vi "HXG2_WriteTDMS.vi"(0 "Air-Liq Cluster":T3 {"Liq Cluster"."Liq TEMP %" min=0.0 max=100.0 step=1.0 format="%#.1f"; "Liq Cluster"."Liq FLOW %" min=0.0 max=100.0 step=1.0 format="%#.1f"; "Liq Cluster"."TLiq °F" min=40.0 max=180.0 step=1.0 format="%#.1f"; "Liq Cluster"."Mdot lbm/hr" min=0.0 max=1000.0 step=1.0 format="%#.1f"; "Air Cluster"."Air TEMP %" min=0.0 max=100.0 step=1.0 format="%#.1f"; "Air Cluster"."Air FLOW %" min=0.0 max=100.0 step=1.0 format="%#.1f"; "Air Cluster"."Tair  °F" min=-5.0 max=100.0 step=1.0 format="%#.1f"; "Air Cluster"."CFMs" min=0.0 max=200.0 step=1.0 format="%#.1f"}, 2 "Save?":bool, 5 "Calcs":T2, 7 "Excel/Elapsed t":dbl[](array[numeric]), 9 "DATA In":T1, 11 "error in":errorcluster, 12 "tdms file":refnum<k34>, 14 "Test Point":i32) -> (4 "tdms file out":refnum<k34>, 15 "error out":errorcluster)   [LabVIEW 2012]
uses:
  Controls/HXG2_AirGly-Cluster.ctl
  Controls/UI/HXG2_UI_ControlSetAir.ctl
  Controls/UI/HXG2_UI_ControlSetGly.ctl
  Controls/HXG2_Calculated.ctl
  Controls/HXG2_AnalogIn.ctl
  HXG2saveTimer.ctl
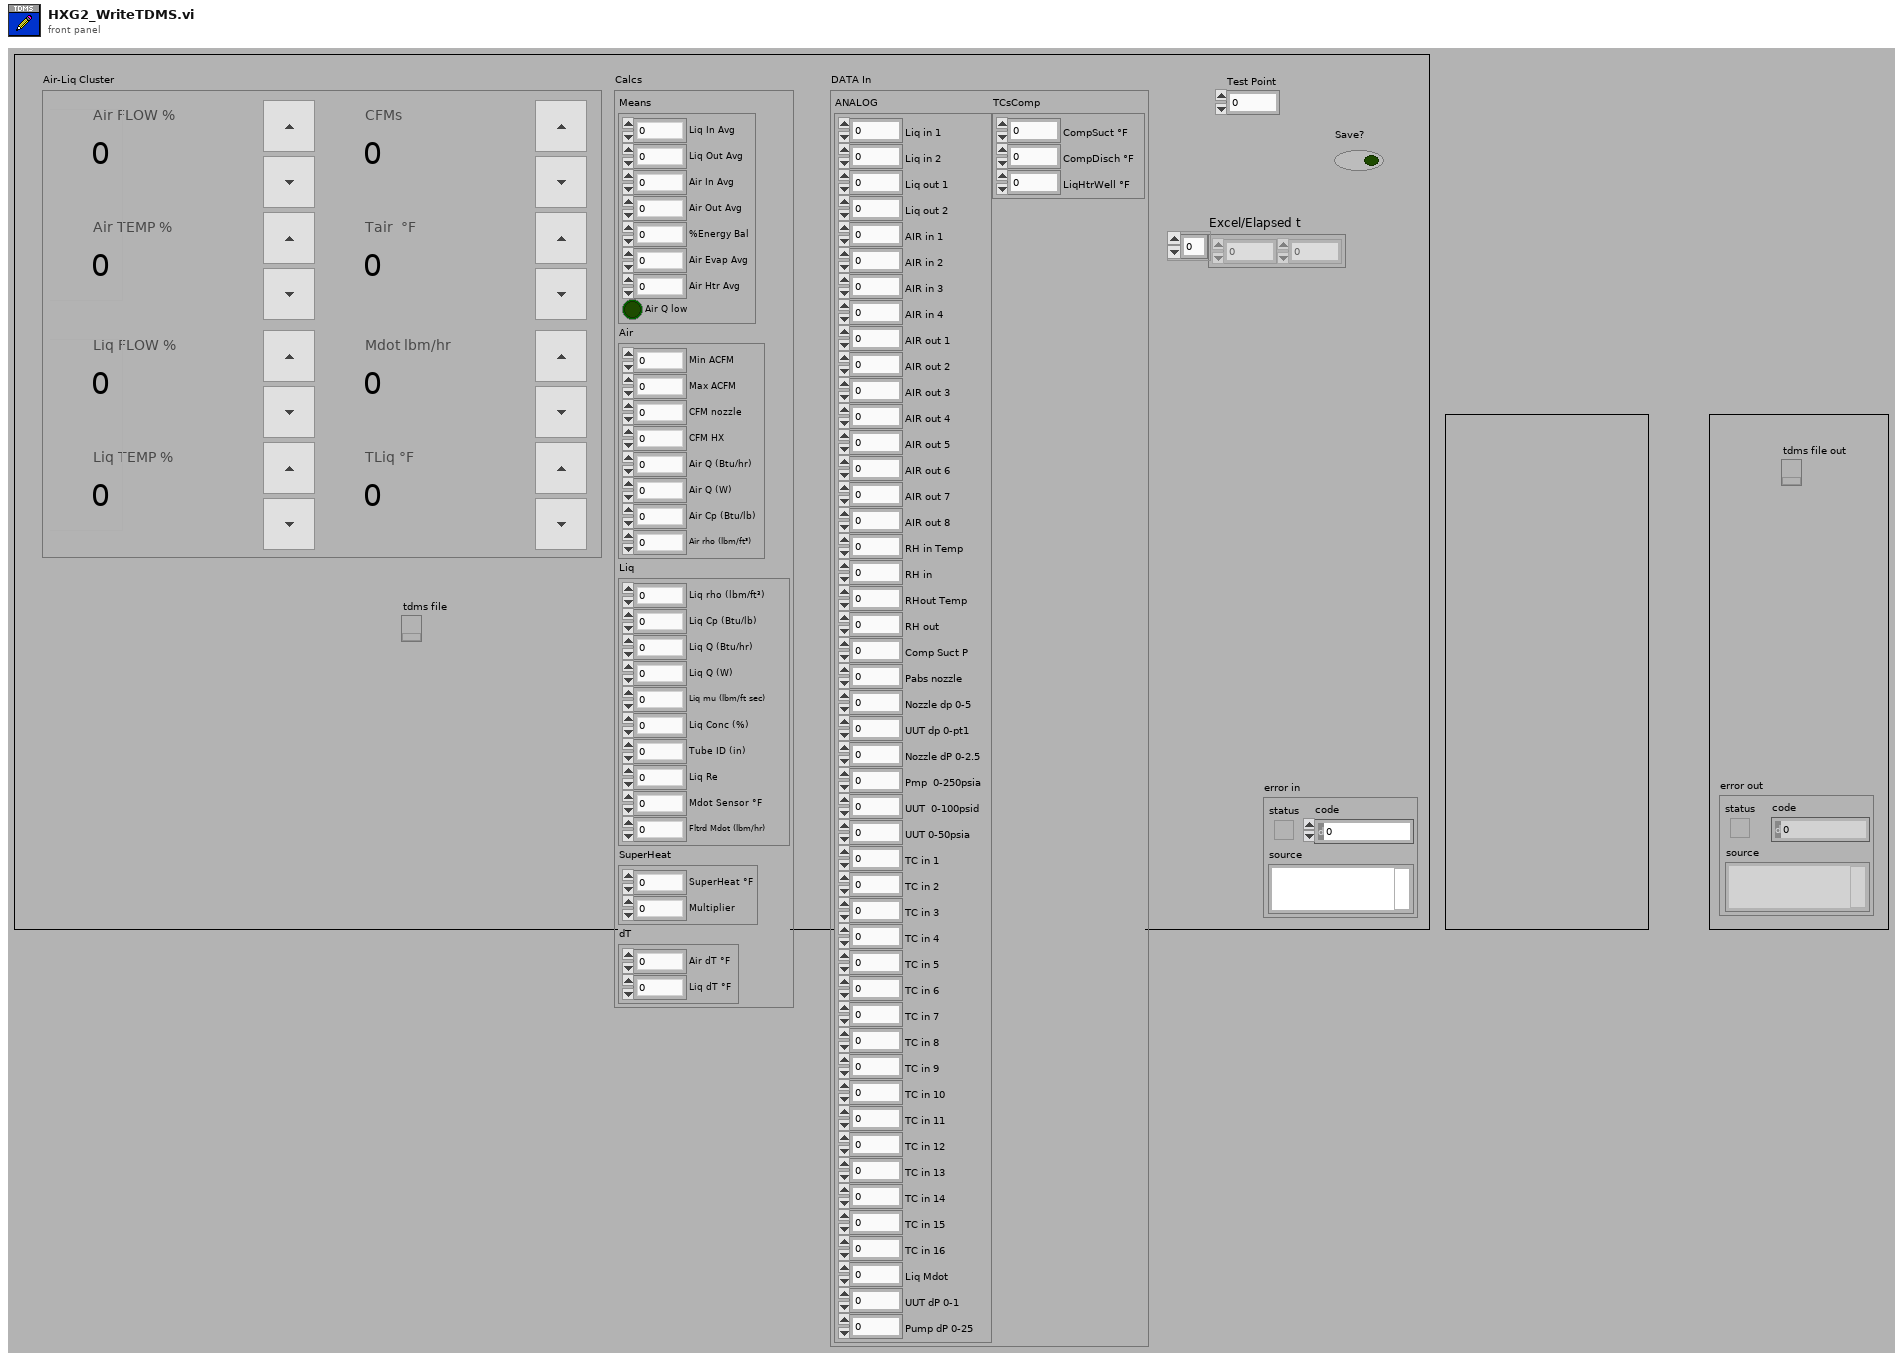
[diagram p1: front panel]
types:
  T1 = typedef "HXG2_AnalogIn.ctl" = cluster{"ANALOG":cluster{"Liq in 1":dbl, "Liq in 2":dbl, "Liq out 1":dbl, "Liq out 2":dbl, "AIR in 1":dbl, "AIR in 2":dbl, "AIR in 3":dbl, "AIR in 4":dbl, "AIR out 1":dbl, "AIR out 2":dbl, "AIR out 3":dbl, "AIR out 4":dbl, "AIR out 5":dbl, "AIR out 6":dbl, "AIR out 7":dbl, "AIR out 8":dbl, "RH in Temp":dbl, "RH in":dbl, "RHout Temp":dbl, "RH out":dbl, "Comp Suct P":dbl, "Pabs nozzle":dbl, "Nozzle dp 0-5":dbl, "UUT dp 0-pt1":dbl, "Nozzle dP 0-2.5":dbl, "Pmp  0-250psia":dbl, "UUT  0-100psid":dbl, "UUT 0-50psia":dbl, "TC in 1":dbl, "TC in 2":dbl, "TC in 3":dbl, "TC in 4":dbl, "TC in 5":dbl, "TC in 6":dbl, "TC in 7":dbl, "TC in 8":dbl, "TC in 9":dbl, "TC in 10":dbl, "TC in 11":dbl, "TC in 12":dbl, "TC in 13":dbl, "TC in 14":dbl, "TC in 15":dbl, "TC in 16":dbl, "Liq Mdot":dbl, "UUT dP 0-1":dbl, "Pump dP 0-25":dbl}, "TCsComp":cluster{"CompSuct °F  ":dbl, "CompDisch °F":dbl, "LiqHtrWell °F":dbl}}
  T2 = typedef "HXG2_Calculated.ctl" = cluster{"Means":cluster{"Liq In Avg":dbl, "Liq Out Avg":dbl, "Air In Avg":dbl, "Air Out Avg":dbl, "%Energy Bal":dbl, "Air Evap Avg":dbl, "Air Htr Avg":dbl, "Air Q low":bool}, "Air":cluster{"Min ACFM":dbl, "Max ACFM":dbl, "CFM nozzle":dbl, "CFM HX":dbl, "Air Q (Btu/hr)":dbl, "Air Q (W)":dbl, "Air Cp (Btu/lb)":dbl, "Air rho (lbm/ft³)":dbl}, "Liq":cluster{"Liq rho (lbm/ft³)":dbl, "Liq Cp (Btu/lb)":dbl, "Liq Q (Btu/hr)":dbl, "Liq Q (W)":dbl, "Liq mu (lbm/ft sec)":dbl, "Liq Conc (%)":dbl, "Tube ID (in)":dbl, "Liq Re":dbl, "Mdot Sensor °F":dbl, "Fltrd Mdot (lbm/hr)":dbl}, "SuperHeat":cluster{"SuperHeat °F":dbl, "Multiplier":dbl}, "dT":cluster{"Air dT °F":dbl, "Liq dT °F":dbl}}
  T3 = typedef "HXG2_AirGly-Cluster.ctl" = cluster{"Air Cluster":T4, "Liq Cluster":T5}
  T4 = typedef "HXG2_UI_ControlSetAir.ctl" = cluster{"Air FLOW %":dbl, "Air TEMP % ":dbl, "CFMs":dbl, "Tair  °F":dbl}
  T5 = typedef "HXG2_UI_ControlSetGly.ctl" = cluster{"Liq FLOW %":dbl, "Liq TEMP % ":dbl, "Mdot lbm/hr":dbl, "TLiq °F":dbl}
  T6 = typedef "HXG2saveTimer.ctl" = enum16{"EvntStrtDurtn", "EvntStrtInterv", "Stop", "Check", "RegStrtInterv", "Add10Durtn", "Take10Durtn"}
  T7 = cluster{"System Setpoints":string[], "Means":string[], "Air Props":string[], "Liq Props":string[], "System Data":string[], "All Temps":string[], "Other Data":string[], "CoilDesigner":string[]}
  T8 = typedef "HXG2_NumDisplayLarge.ctl" = dbl
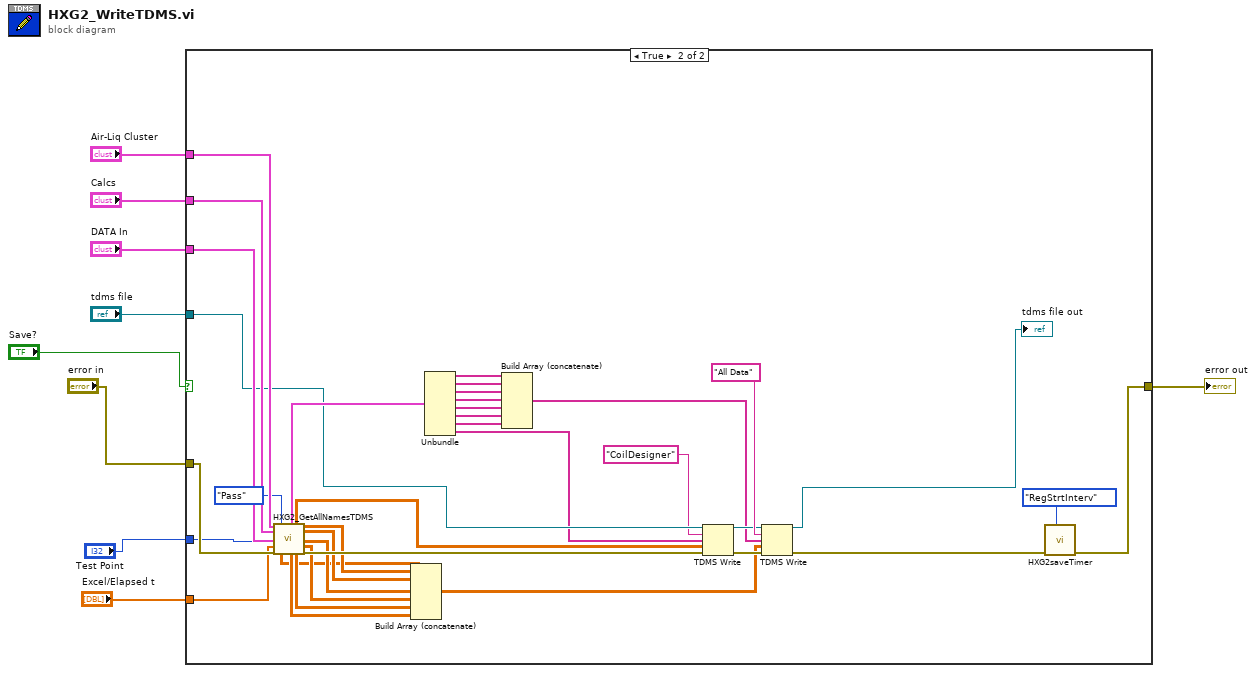
[diagram p0: block diagram]
diagram:
  n1 = case shown="True" "Save?" {
    tunnel: [w10 w32] -> w9
    tunnel: "Air-Liq Cluster" -> [_ w43]
    tunnel: "Calcs" -> [_ w42]
    tunnel: "DATA In" -> [_ w41]
    tunnel: "tdms file" -> [_ w36]
    tunnel: "error in" -> [w10 w35]
    tunnel: "Test Point" -> [_ w14]
    tunnel: "Excel/Elapsed t" -> [_ w13]
    frame False {
    }
    frame True {
      n2 = call "HXG2_GetAllNamesTDMS.vi"("Air-Liq Cluster"=w43, "Calcs"=w42, "DATA In"=w41, "Test Point"=w14, "Excel/Elapsed t"=w13, "error in (no error)"=w35, "Control"=enum16{"Initialize", "Pass"}."Pass") -> ("SetPoints"=w25:dbl[][], "Cluster"=w37:T7, "Other Data"=w26:dbl[][], "For CoilDesigner"=w38:T8[][], "All Temps"=w27:dbl[][], "Means"=w31:dbl[][], "Air Props"=w30:dbl[][], "Liq Props"=w29:dbl[][], "Syst Data"=w28:dbl[][], "error out"=w40:errorcluster)  [unwired: 3 in]
      n3 = Build Array (concatenate)(w25, w31, w30, w29, w28, w27, w26) -> (w24:dbl[][])
      n4 = Unbundle(w37) -> ("System Setpoints"=w22:string[], "Means"=w21:string[], "Air Props"=w20:string[], "Liq Props"=w19:string[], "System Data"=w18:string[], "All Temps"=w17:string[], "Other Data"=w16:string[], "CoilDesigner"=w23:string[])
      n5 = Build Array (concatenate)(w22, w21, w20, w19, w18, w17, w16) -> (w15:string[])
      n6 = TDMS Write(0:w36, 5:"CoilDesigner", 7:w23, 9:w38, 11:w40) -> (4:w44:refnum<k34>, 15:w45:errorcluster)  [unwired: 1 in, 2 out]
      n7 = TDMS Write(0:w44, 5:"All Data", 7:w15, 9:w24, 11:w45) -> (4:→"tdms file out":refnum<k34>, 15:w12:errorcluster)  [unwired: 1 in, 2 out]
      n8 = call "HXG2saveTimer.vi"("SaveTimerFGV"=HXG2saveTimer."RegStrtInterv", "error in (no error)"=w12) -> ("error out"=w32:errorcluster)  [unwired: 5 in, 4 out]
    }
  }
  "error out" <- w9
